vi "showError.vi"(3 "message":string, 5 "Error IN":errorcluster) -> (2 "Error OUT":errorcluster)   [LabVIEW 2010]
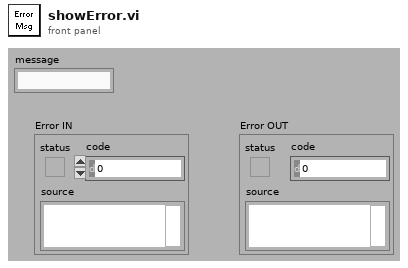
[diagram p1: front panel]
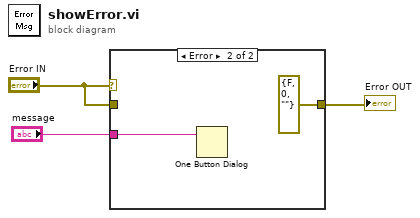
[diagram p0: block diagram]
diagram:
  n1 = case shown="Error" "Error IN" {
    tunnel: [w4 errorcluster {"status"=FALSE, "code"=0, "source"=""} ("Error OUT")] -> w3
    tunnel: "Error IN" -> [w4 _]
    tunnel: "message" -> [_ w5]
    frame No Error {
    }
    frame Error {
      n2 = One Button Dialog(message=w5) -> ()  [unwired: 1 in, 1 out]
    }
  }
  "Error OUT" <- w3
